vi "SyncronousLockinProcessing.vi"() -> ()   [LabVIEW 2016]
doc: "Syncronous lock-in processing allows for simultaneous processing of multiple sine frequencies, auto-fill option for data channels and rates (for that one should have couple of strings in the s0*.txt settings file such as:\n\nLockin_channels = channel_name, channel_name,...\nLockin_points = points_per_sine_wave, points_per_sine_wave,...\n\nlisting all lock-in data channels and sine wave rates in a s0*.tdms file.\n\nI also added finite impulse response low-pass filter alternative in addition to old infinite impulse response one.\n\nThere's a new app in the same folder \\NHMFL\\LANL\\Applications\\PulsedMagnetDAQ\nnamed Filter design.vi, which allows one to visualize filter's time and frequency response with given settings."
uses:
  Libraries/SoftwareLockin/CH_name_pts_phase.ctl
  Libraries/SoftwareLockin/Syncronous Lockin Settings.ctl
panel:
  in  "Auto fill channels":bool
  in  "Fiter selector":T1(tab)=enum."Infinite response"
  in  "IIR Low-pass filter":T2={"Clip IIR filter ramps, 1/Fc"=1.0, "Two-pass & flip"=TRUE, "IIR filter specifications"={"Topology"=enum."Butterworth", "Type"=enum."Lowpass", "Order"=1, "Lower Fc"=5000.0, "Upper Fc"=200.0, "PB Ripple"=1.0, "SB Attenuation"=60.0}} {"IIR filter specifications"."PB Ripple" format="%0.2f"; "IIR filter specifications"."Lower Fc" format="%0.2p"; "IIR filter specifications"."SB Attenuation" format="%0.2f"; "IIR filter specifications"."Upper Fc" format="%0.2p"}
  in  "FIR Low-pass filter":T3={"Clip IIR filter ramps, 1/Fc"=2.0, "Two-pass & flip"=TRUE, "FIR filter specifications"={"Topology"=enum."Windowed FIR", "Type"=enum."Lowpass", "#Taps"=50, "Lower PB"=2000.0, "Upper PB"=0.0, "Lower SB"=4000.0, "Upper SB"=0.0}, "optional FIR filter\n specifications"={"PB Gain"=-3.0, "SB Gain"=-60.0, "Scale"=TRUE, "Window"=enum."Hanning"}} {"optional FIR filter\n specifications"."SB Gain" format="%.2p"; "optional FIR filter\n specifications"."PB Gain" format="%.2p"; "FIR filter specifications"."Lower SB" format="%0.2p"; "FIR filter specifications"."Upper SB" format="%0.2p"; "FIR filter specifications"."Lower PB" format="%0.2p"; "FIR filter specifications"."Upper PB" format="%0.2p"; "Clip IIR filter ramps, 1/Fc" format="%#_6p"}
  in  "Lock-in settings":T4={"Averaging period, s"=0.0, "Output Representation"=enum."Real/Imaginary", "Output value"=enum."RMS", "Phase delay, points"=0} {"Averaging period, s" format="%#_6p"}
  in  "Channel info":T5[](array[typedef]) caption="Channel                   pts per sine    phase"
  in  "Overwrite\nclock, Hz":dbl=nan format="%#_20p"
  in  "DOWN":bool
  in  "UP":bool
  out "error out":errorcluster={"status"=FALSE, "code"=1800, "source"="Start or end time rounded to nearest value in Get Waveform Subset.VI."}
  in  "Bin size":dbl=0.05 format="%.2f"
  in  "Save binned ASCII":bool
  out "In-phase/Amplitude":waveform(dbl)[](graph)
  out "XY Graph":cluster{"Y":dbl[], "Y":dbl[]}[](graph)
  out "Out-of-phase/Phase angle":waveform(dbl)[](graph)
  in  "Done":bool
  in  "Manual\nPhase":dbl(slide) scale=-180.0..180.0
  in  "Manual phase adjustment":bool=TRUE
  in  "Save column names":bool
  in  "Save ASCII file":bool
  in  "Interpolate to X":bool=TRUE
  in  "X column name":string="Field_fixed"
  out "CH lengh":u64=1960400
  in  "group name":string="Untitled"
  in  "error in (no error)":errorcluster
  in  "Data file path":path=path "C:/Data/October_2012/100112/s004_100112.tdms"
  in  "Raw chunk size":i64=500000 format="%.0p"
  # "Soft lock-in"
  # "F.F.Balakirev"
  # "No filter will be applied"
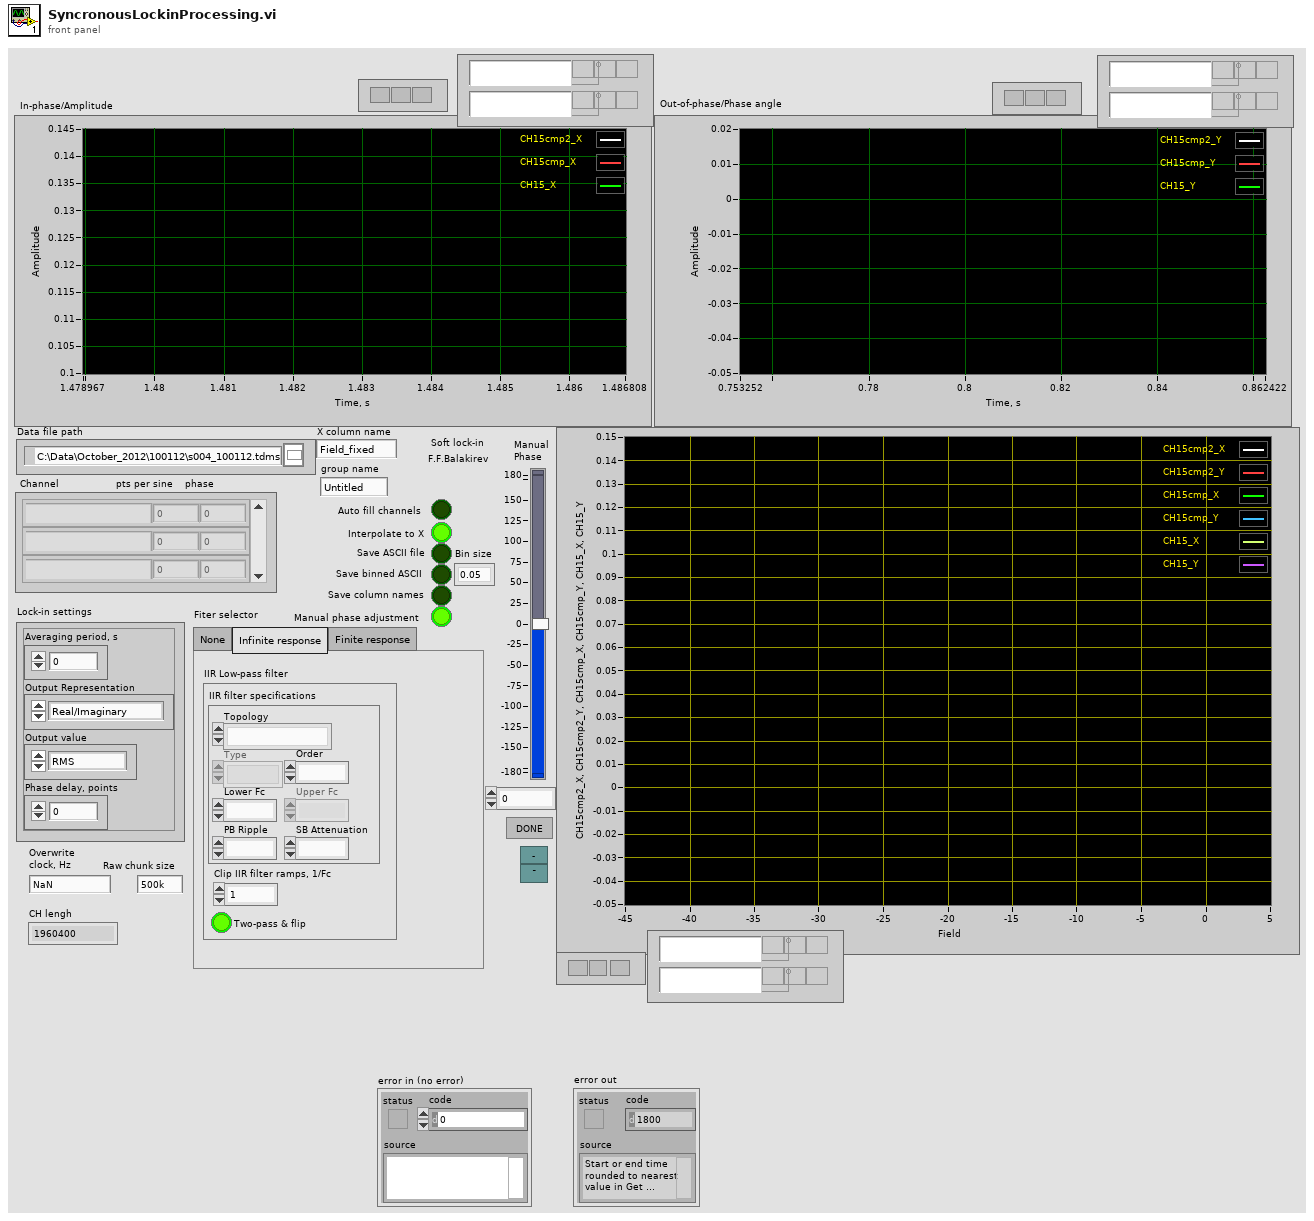
[diagram p1: front panel]
types:
  T1 = enum32{"None", "Infinite response", "Finite response"}
  T2 = cluster{"Clip IIR filter ramps, 1/Fc":dbl, "Two-pass & flip":bool, "IIR filter specifications":cluster{"Topology":enum16{"Off", "Butterworth", "Chebyshev", "Inverse Chebyshev", "Elliptic", "Bessel"}, "Type":enum16{"Lowpass", "Highpass", "Bandpass", "Bandstop"}, "Order":i32, "Lower Fc":dbl, "Upper Fc":dbl, "PB Ripple":dbl, "SB Attenuation":dbl}}
  T3 = cluster{"Clip IIR filter ramps, 1/Fc":dbl, "Two-pass & flip":bool, "FIR filter specifications":cluster{"Topology":enum16{"Off", "FIR by Specification", "Equi-ripple FIR", "Windowed FIR"}, "Type":enum16{"Lowpass", "Highpass", "Bandpass", "Bandstop"}, "#Taps":i32, "Lower PB":dbl, "Upper PB":dbl, "Lower SB":dbl, "Upper SB":dbl}, "optional FIR filter\n specifications":cluster{"PB Gain":dbl, "SB Gain":dbl, "Scale":bool, "Window":enum16{"None", "Hanning", "Hamming", "Triangular", "Blackman", "Exact Blackman", "Blackman-Harris", "Kaiser-Bessel", "Flat Top"}}}
  T4 = typedef "Syncronous Lockin Settings.ctl" = cluster{"Averaging period, s":dbl, "Output Representation":enum16{"Real/Imaginary", "Polar"}, "Output value":enum16{"Amplitude", "RMS", "Peak-to-Peak"}, "Phase delay, points":i32}
  T5 = typedef "CH_name_pts_phase.ctl" = cluster{"Channel":string, "pts per sine wave":i32, "Phase":dbl}
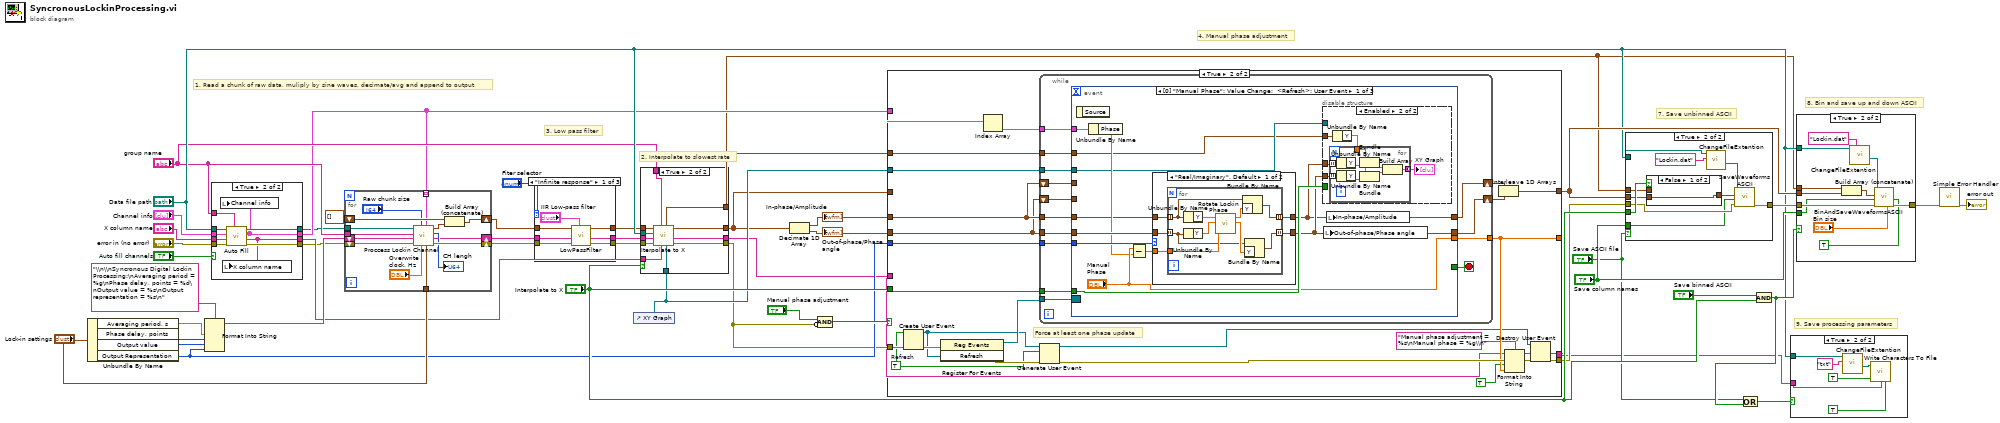
[diagram p0: block diagram]
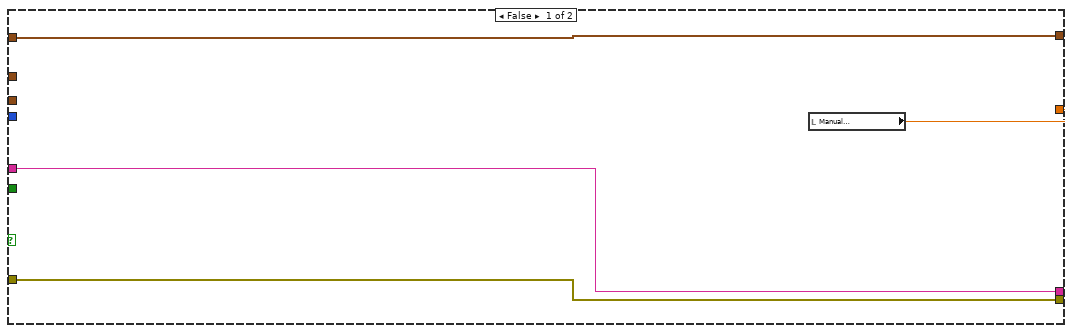
[diagram p5: hidden frame]
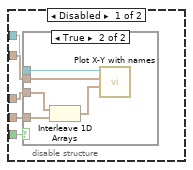
[diagram p6: hidden frame]
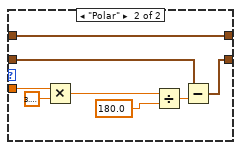
[diagram p8: hidden frame]
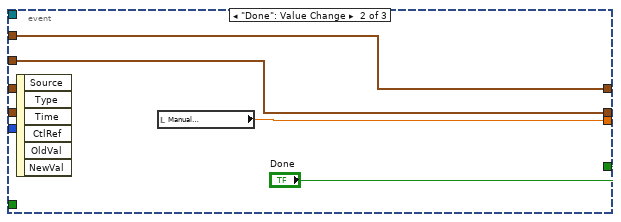
[diagram p9: hidden frame]
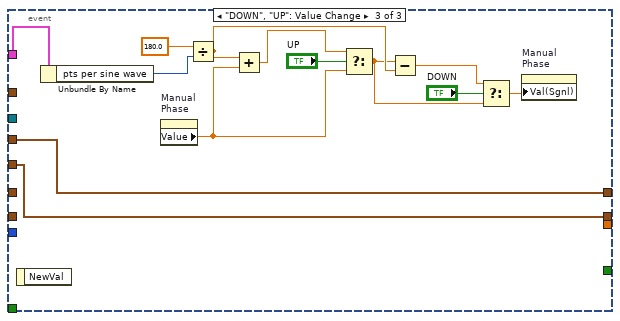
[diagram p10: hidden frame]
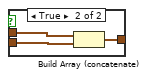
[diagram p12: hidden frame]
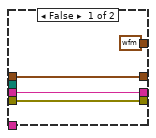
[diagram p13: hidden frame]
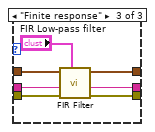
[diagram p15: hidden frame]
diagram:
  # "9. Save processing parameters"
  # "8. Bin and save up and down ASCII"
  # "7. Save unbinned ASCII"
  # "4. Manual phase adjustment"
  # "2. Interpolate to slowest rate"
  # "3. Low pass filter"
  # "1. Read a chunk of raw data, muliply by sine waves, decimate/avg and append to output"
  n1 = Unbundle By Name("Lock-in settings") -> ("Averaging period, s"=w27:dbl, "Phase delay, points"=w26:i32, "Output value"=w25:enum16{"Amplitude", "RMS", "Peak-to-Peak"}, "Output Representation"=w24:enum16{"Real/Imaginary", "Polar"})
  n2 = Format Into String(format string="\\n\\nSyncronous Digital Lockin Processing:\nAveraging period = %g\nPhase delay, points = %d\nOutput value = %s\nOutput representation = %s\n", w27, w26, w25, w24) -> (resulting string=w23:string)  [unwired: 2 in, 1 out]
  n3 = case shown="True" "Auto fill channels" {
    tunnel: "Data file path" -> [w47 w59]
    tunnel: "Channel info" -> [w50 w58]
    tunnel: "group name" -> [_ w57]
    tunnel: [w50 w53] -> w17
    tunnel: "X column name" -> [w49 w52]
    tunnel: [w49 w51] -> w15
    tunnel: "error in (no error)" -> [w48 w56]
    tunnel: [w48 w55] -> w13
    tunnel: [w47 w54] -> w12
    frame False {
    }
    frame True {
      n4 = call "Auto Fill.vi"("group name"=w57, "Error In"=w56, "X column name"=w52, "Channel info"=w58, "Data file path"=w59) -> ("Error Out"=w55:errorcluster, "X column name out"=w51:string, "Channel info out"=w53:T5[], "Data file path out"=w54:path)  [unwired: 3 in]
      n5 = local write "Channel info"(w53) -> ()
      n6 = local write "X column name"(w51) -> ()
    }
  }
  n7 = for {
    tunnel: w12 -> [w71]
    tunnel: "group name" -> [w70]
    tunnel: w17 -> [w67] mode=indexing
    shift-right: [w69] -> w9
    shift-left: waveform(dbl)[] [] -> [w68]
    shift-right: [w72] -> w7
    shift-left: w13 -> [w73]
    tunnel: "Lock-in settings" -> [w66]
    shift-right: [w61] -> w8
    shift-left: w23 -> [w60]
    n8 = call "Proccess Lockin Channel.vi"("Lock-in settings"=w66, "Channel info"=w67, "Overwrite\nclock, Hz"="Overwrite\nclock, Hz", "Raw chunk size"="Raw chunk size", "error in (no error)"=w73, "Settings"=w60, "group name"=w70, "Data file path"=w71) -> ("error out"=w72:errorcluster, "Settings out"=w61:string, "Channel Length"=→"CH lengh":u64, "signal(s) out"=w64:waveform(dbl)[])
    n9 = Build Array (concatenate)(w68, w64) -> (w69:waveform(dbl)[])
  }
  n10 = case shown="\"Infinite response\"" "Fiter selector" {
    tunnel: w9 -> [w80 w83 w86]
    tunnel: [w79 w83 w90] -> w5
    tunnel: w8 -> [w78 w82 w89]
    tunnel: [w77 w82 w88] -> w3
    tunnel: w7 -> [w75 w81 w85]
    tunnel: [w74 w81 w84] -> w1
    frame "Infinite response" {
      n11 = call "LowPassFilter.vi"("Low-pass filter"="IIR Low-pass filter", "error in (no error)"=w75, "Settings"=w78, "signal(s) in"=w80) -> ("error out"=w74:errorcluster, "Settings out"=w77:string, "signal(s) out"=w79:waveform(dbl)[])  [unwired: 1 in, 4 out]
    }
    frame "None", Default {
    }
    frame "Finite response" {
      n12 = call "FIR Filter.vi"("FIR Low-pass filter"="FIR Low-pass filter", "error in (no error)"=w85, "Settings"=w89, "signal(s) in"=w86) -> ("error out"=w84:errorcluster, "Settings out"=w88:string, "signal(s) out"=w90:waveform(dbl)[])  [unwired: 4 in, 1 out]
    }
  }
  n13 = control-ref of="XY Graph"() -> (w11:refnum<vi>)
  n14 = case shown="True" "Interpolate to X" {
    tunnel: w5 -> [w93 w103]
    tunnel: w1 -> [w94 w104]
    tunnel: "Data file path" -> [_ w101]
    tunnel: [w94 w105] -> w2
    tunnel: [waveform(sgl) {"t0"=timestamp(0 s since 1904-01-01), "dt"=1.0, "Y"=[]} ("data type") w102] -> w10
    tunnel: [w93 w95] -> w6
    tunnel: "group name" -> [_ w98]
    tunnel: w3 -> [w91 w100]
    tunnel: [w91 w99] -> w4
    tunnel: w15 -> [_ w97]
    tunnel: w11 -> [_ w96]
    frame False {
    }
    frame True {
      n15 = call "Iterpolate to X.vi"("XY Graph Ref"=w96, "X column name"=w97, "group name"=w98, "error in (no error)"=w104, "Settings"=w100, "Data file path"=w101, "signal(s) in"=w103) -> ("error out"=w105:errorcluster, "Settings out"=w99:string, "Signals out"=w95:waveform(dbl)[], "X waveform out"=w102:waveform(dbl))  [unwired: 1 in]
    }
  }
  n16 = Decimate 1D Array(w6) -> (w35:waveform(dbl)[], w34:waveform(dbl)[])
  "Out-of-phase/Phase angle" <- w34
  "In-phase/Amplitude" <- w35
  n17 = Compound Arithmetic op=AND("Manual phase adjustment", invert w2) -> (w32:bool)
  n18 = case shown="True" w32 {
    tunnel: w6 -> [w109 _]
    tunnel: w24 -> [_ w135]
    tunnel: w35 -> [_ w134]
    tunnel: w34 -> [_ w133]
    tunnel: "Interpolate to X" -> [_ w132]
    tunnel: w10 -> [_ w131]
    tunnel: [w109 w128] -> w45
    tunnel: w2 -> [w108 w127]
    tunnel: [w108 w111] -> w30
    tunnel: [w107 w118] -> _
    tunnel: w17 -> [_ w121]
    tunnel: w4 -> [w106 w116]
    tunnel: [w106 w115] -> w22
    tunnel: w11 -> [_ w113]
    frame False {
      n19 = local read "Manual\nPhase"() -> (w107:dbl)
    }
    frame True {
      w122 = TRUE  # Refresh
      # "Force at least one phase update"
      n20 = Create User Event(user event datatype=w122, error in=w127) -> (user event=w123:refnum<user-event>, error out=w126:errorcluster)
      n21 = register-events(error in=w126, w123) -> (reference out=w124:refnum<event-registration>, error out=w125:errorcluster)  [unwired: 1 in]
      n22 = Index Array(array=w121) -> (element=w120:T5)  [unwired: 1 in]
      n23 = while {
        tunnel: w134 -> [w148]
        tunnel: w133 -> [w147]
        tunnel: w135 -> [w146]
        shift-right: [w145] -> w130
        shift-left: w134 -> [w143]
        shift-right: [w144] -> w129
        shift-left: w133 -> [w142]
        tunnel: w132 -> [w141]
        tunnel: w131 -> [w140]
        tunnel: w124 -> [w139]
        tunnel: [w138] -> w118
        tunnel: w120 -> [w137]
        tunnel: w113 -> [w136]
        stop <- w149 stop-if-true
        n24 = event shown="[0] \"Manual Phase\": Value Change;  <Refresh>: User Event" {
          selector: w139 -> [_ _ _]
          dyn-events: _ -> [_ _ _]
          timeout: _ -> [_ _ _]
          tunnel: [_ "Done" _] -> w149
          tunnel: w148 -> [w152 _ _]
          tunnel: w147 -> [w160 _ _]
          tunnel: w146 -> [w161 _ _]
          tunnel: [w158 w208 w213] -> w144
          tunnel: [w151 w209 w214] -> w145
          tunnel: w143 -> [_ w209 w214]
          tunnel: w142 -> [_ w208 w213]
          tunnel: w141 -> [w159 _ _]
          tunnel: w140 -> [w150 _ _]
          tunnel: ["Manual\nPhase" w207 _] -> w138
          tunnel: w137 -> [w155 _ w211]
          tunnel: w136 -> [w153 _ _]
          event "Manual\nPhase": Value Change; User Event {
            n25 = event-data() -> ()  [unwired: 2 out]
            n26 = Unbundle By Name(w155) -> ("Phase"=w154:dbl)
            n27 = Subtract(x="Manual\nPhase", y=w154) -> (x-y=w157:dbl)
            n28 = case shown="\"Real/Imaginary\", Default" w161 {
              tunnel: w152 -> [w189 w206]
              tunnel: w160 -> [w188 w205]
              tunnel: w157 -> [w187 w202]
              tunnel: [w186 w204] -> w158
              tunnel: [w185 w206] -> w151
              frame "Real/Imaginary", Default {
                n29 = for {
                  tunnel: w189 -> [w194] mode=indexing
                  tunnel: w188 -> [w192] mode=indexing
                  tunnel: w187 -> [w196]
                  tunnel: [w191] -> w186 mode=indexing
                  tunnel: [w190] -> w185 mode=indexing
                  n30 = Unbundle By Name(w192) -> ("Y"=w197:dbl[])
                  n31 = Unbundle By Name(w194) -> ("Y"=w198:dbl[])
                  n32 = call "Rotate Lockin Phase.vi"("Phase"=w196, "Array Y in"=w197, "Array X in"=w198) -> ("Array Y out"=w193:dbl[], "Array X out"=w195:dbl[])  [unwired: 7 out]
                  n33 = Bundle By Name(cluster=w194, "Y"=w195) -> (w190:waveform(dbl))
                  n34 = Bundle By Name(cluster=w192, "Y"=w193) -> (w191:waveform(dbl))
                }
              }
              frame "Polar" {
                n35 = Multiply(x=w202, y=3.141592653589793) -> (x*y=w201:dbl)
                n36 = Divide(x=w201, y=180.0) -> (x/y=w200:dbl)
                n37 = Subtract(x=w205, y=w200) -> (x-y=w204:waveform(dbl)[])
              }
            }
            n38 = disable-structure shown="Enabled" {
              disable-tunnel: w159 -> [w166 _]
              disable-tunnel: w150 -> [w165 w174]
              disable-tunnel: w151 -> [w164 w176]
              disable-tunnel: w158 -> [w163 w175]
              disable-tunnel: w153 -> [w162 _]
              frame Disabled {
                n39 = case shown="True" w166 {
                  tunnel: w165 -> [_ w171]
                  tunnel: w164 -> [_ w168]
                  tunnel: w163 -> [_ w170]
                  tunnel: w162 -> [_ w167]
                  frame False {
                  }
                  frame True {
                    n40 = Interleave 1D Arrays(w168, w170) -> (w169:waveform(dbl)[])
                    n41 = call "Plot X-Y with names.vi"("Y columns"=w169, "X column"=w171, "XY Graph Ref"=w167) -> ()  [unwired: 7 in, 2 out]
                  }
                }
              }
              frame Enabled {
                n42 = Unbundle By Name(w174) -> ("Y"=w173:dbl[])
                n43 = for {
                  tunnel: w176 -> [w184] mode=indexing
                  tunnel: w175 -> [w183] mode=indexing
                  tunnel: w173 -> [w180]
                  tunnel: [w177] -> w172 mode=concatenating
                  n44 = Unbundle By Name(w184) -> ("Y"=w182:dbl[])
                  n45 = Unbundle By Name(w183) -> ("Y"=w181:dbl[])
                  n46 = Bundle("Y"=w180, "Y"=w182) -> (w179:cluster{"Y":dbl[], "Y":dbl[]})  [unwired: 1 in]
                  n47 = Bundle("Y"=w180, "Y"=w181) -> (w178:cluster{"Y":dbl[], "Y":dbl[]})  [unwired: 1 in]
                  n48 = Build Array(w179, w178) -> (w177:cluster{"Y":dbl[], "Y":dbl[]}[])
                }
                "XY Graph" <- w172
              }
            }
            n49 = local write "Out-of-phase/Phase angle"(w158) -> ()
            n50 = local write "In-phase/Amplitude"(w151) -> ()
          }
          event "Done": Value Change {
            n51 = event-data() -> ()  [unwired: 7 out]
            n52 = local read "Manual\nPhase"() -> (w207:dbl)
          }
          event "DOWN", "UP": Value Change {
            n53 = event-data() -> ()  [unwired: 2 out]
            n54 = Unbundle By Name(w211) -> ("pts per sine wave"=w212:i32)
            n55 = property on="Manual\nPhase" class="Slide (strict)"() -> ("Value"=w215:dbl)  [unwired: 2 in, 2 out]
            n56 = Divide(x=180.0, y=w212) -> (x/y=w220:dbl)
            n57 = Add(x=w220, y=w215) -> (x+y=w222:dbl)
            n58 = Select(t=w222, s="UP", f=w215) -> (s? t:f=w216:dbl)
            n59 = Subtract(x=w216, y=w220) -> (x-y=w219:dbl)
            n60 = Select(t=w219, s="DOWN", f=w216) -> (s? t:f=w217:dbl)
            n61 = property on="Manual\nPhase" class="Slide (strict)"("Val(Sgnl)"=w217) -> ()  [unwired: 2 in, 2 out]
          }
        }
      }
      n62 = Generate User Event(user event=w123, event data cluster=w122, error in=w125) -> (user event out=w110:refnum<user-event>, error out=w119:errorcluster)  [unwired: 1 in]
      n63 = Interleave 1D Arrays(w130, w129) -> (w128:waveform(dbl)[])
      n64 = Format Into String(format string="Manual phase adjustment = %s\nManual phase = %g\\n", initial string=w116, error in=w119, TRUE ("input 1"), w118) -> (resulting string=w115:string, error out=w112:errorcluster)
      n65 = Destroy User Event(user event=w110, error in=w112) -> (error out=w111:errorcluster)
    }
  }
  n66 = case shown="True" "Save ASCII file" {
    tunnel: w30 -> [w224 w226]
    tunnel: w45 -> [_ w228]
    tunnel: "Interpolate to X" -> [_ w234]
    tunnel: w10 -> [_ w233]
    tunnel: "Data file path" -> [_ w232]
    tunnel: [w224 w230] -> w44
    tunnel: "Save column names" -> [_ w225]
    frame False {
    }
    frame True {
      n67 = case shown="False" w234 {
        tunnel: w233 -> [_ w238]
        tunnel: w228 -> [w235 w237]
        tunnel: [w235 w236] -> w227
        frame False {
        }
        frame True {
          n68 = Build Array (concatenate)(w238, w237) -> (w236:waveform(dbl)[])
        }
      }
      n69 = call "ChangeFileExtention.vi"("New Extention"="Lockin.dat", "Path"=w232) -> ("Path with new extension"=w229:path)  [unwired: 1 in, 8 out]
      n70 = call "SaveWaveformsASCII.vi"("Error In"=w226, "Save column names"=w225, "Waveforms"=w227, "File"=w229) -> ("Error Out"=w230:errorcluster)  [unwired: 4 in, 3 out]
    }
  }
  n71 = And(x="Save binned ASCII", y="Interpolate to X") -> (x .and. y?=w40:bool)
  n72 = Compound Arithmetic op=OR("Save ASCII file", w40) -> (w38:bool)
  n73 = case shown="True" w38 {
    tunnel: "Data file path" -> [_ w244]
    tunnel: w22 -> [_ w239]
    frame False {
    }
    frame True {
      n74 = call "ChangeFileExtention.vi"("New Extention"="txt", "Path"=w244) -> ("Path with new extension"=w242:path)  [unwired: 1 in, 8 out]
      n75 = call <vilib>:"Write Characters To File.vi"("convert eol? (no:F)"=TRUE, "append to file? (new file:F)"=TRUE, "character string"=w239, "file path (dialog if empty)"=w242) -> ()  [unwired: 2 out]
    }
  }
  n76 = case shown="True" w40 {
    tunnel: w44 -> [w245 w249]
    tunnel: w45 -> [_ w251]
    tunnel: w10 -> [_ w256]
    tunnel: "Data file path" -> [_ w255]
    tunnel: [w245 w253] -> w37
    tunnel: "Save column names" -> [_ w248]
    frame False {
    }
    frame True {
      n77 = Build Array (concatenate)(w256, w251) -> (w250:waveform(dbl)[])
      n78 = call "ChangeFileExtention.vi"("New Extention"="Lockin.dat", "Path"=w255) -> ("Path with new extension"=w252:path)  [unwired: 1 in, 8 out]
      n79 = call "BinAndSaveWaveformsASCII.vi"("transpose? (no:F)"=TRUE, "X step"="Bin size", "error in"=w249, "Save column names"=w248, "Y waveforms in"=w250, "file (use dialog)"=w252) -> ("error out"=w253:errorcluster)  [unwired: 3 in, 2 out]
    }
  }
  n80 = call <vilib>:"Simple Error Handler.vi"("error in (no error)"=w37) -> ("error out"=→"error out":errorcluster)  [unwired: 1 in, 7 out]
